vi "torquesptohexstrings.vi"(11 "torque value":sgl) -> (3 "String out":string)   [LabVIEW 2019]
panel:
  in  "Register number":u16=22000
  out "data string":string
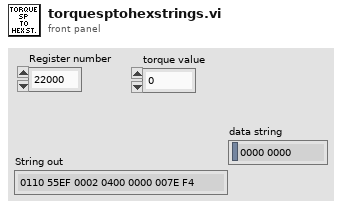
[diagram p1: front panel]
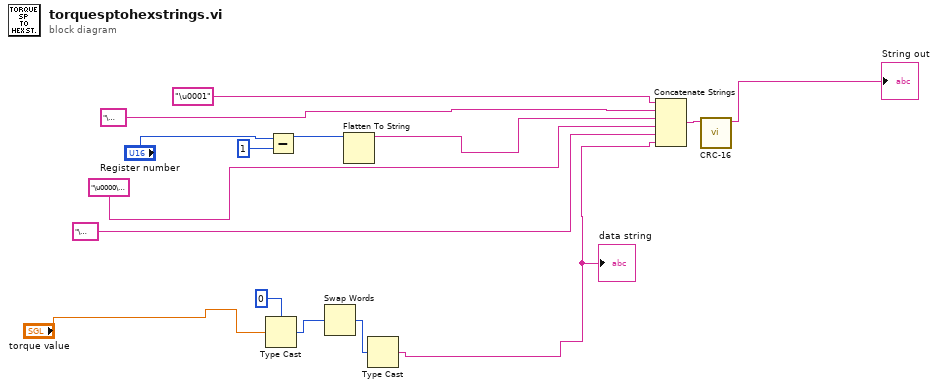
[diagram p0: block diagram]
diagram:
  n1 = Type Cast(type=u32 0 ("Register number 2"), x="torque value") -> (*(type *) &x=w3:u32)
  n2 = Subtract(x="Register number", y=u16 1) -> (x-y=w7:u16)
  n3 = Swap Words(1:w3) -> (0:w2:u32)
  n4 = Flatten To String(anything=w7) -> (data string=w6:string)  [unwired: 3 in, 2 out]
  n5 = Type Cast(x=w2) -> (*(type *) &x=w1:string)  [unwired: 1 in]
  "data string" <- w1
  n6 = Concatenate Strings("\u0001" ("Address of the Slave in Hex"), "\u0010" ("Function Code in Hex(Write Multiple Registers)"), w6, "\u0000\u0002" ("Number of registers(2bytes-4hexdigits)"), "\u0004" ("string"), w1) -> (w11:string)
  n7 = call "CRC-16.vi"("String in"=w11) -> ("String out"=→"String out":string)  [unwired: 8 in, 2 out]
